vi "ReadMultiTofv2.vi"(6 "Attempts":i32=1, 7 "Relays":tag[](array[tag])=["B/DIO0", "B/DIO1", "B/DIO2", "B/DIO3"], 8 "error in":errorcluster, 10 "I2C Channel":u8=1) -> (0 "error out":errorcluster, 1 "ToF Online":bool[](array[boolean]), 2 "ToF Details":T1[](array[typedef]) {"I2C Slave Address" format="%02x"})   [LabVIEW 2017]
uses:
  <vilib>/myRIO/Common/Instrument Driver Framework/myRIO v1.0/DIO/typedefs/DIO Channels Enum.ctl
  <vilib>/myRIO/Common/Instrument Driver Framework/myRIO v1.0/DIO/typedefs/DIO Channels List.ctl
  <vilib>/myRIO/Common/Instrument Driver Framework/Utilities/typedefs/Generic FPGA Reference.ctl
  <vilib>/myRIO/Common/Instrument Driver Framework/Utilities/typedefs/myRIO v1.0 Reference.ctl
  <vilib>/myRIO/Common/Instrument Driver Framework/Utilities/typedefs/Hardware Version Enum.ctl
  <vilib>/myRIO/Common/Instrument Driver Framework/Utilities/typedefs/myRIO Generic Hardware Reference.ctl
  <vilib>/myRIO/Instrument Drivers/Onboard IO/DIO/typedefs/DIO Reference.ctl
  <vilib>/myRIO/Instrument Drivers/Onboard IO/DIO/DIO.lvlib
  <vilib>/myRIO/Instrument Drivers/Onboard IO/DIO/vis/myRIO DIO Open.xnode
  <vilib>/myRIO/Common/Instrument Driver Framework/myRIO v1.0/DIO/vis/myRIO v1.1 Open DIO.vi
  <vilib>/userdefined/High Color/nirio_resource_hc.ctl
  Sensors/Time of Flight - VL6180/VL6180 Resource.ctl
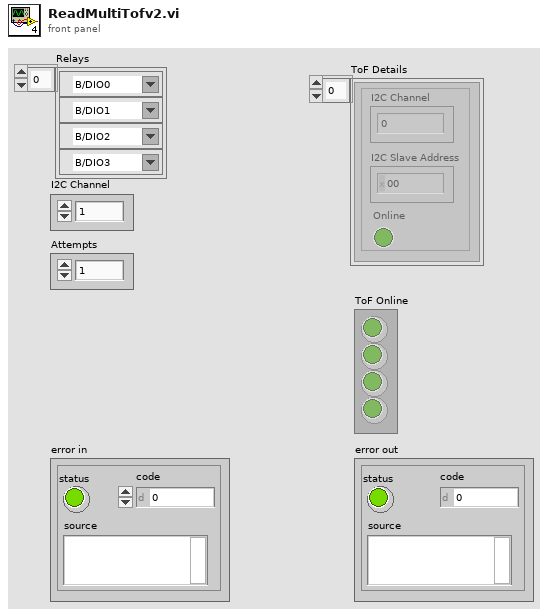
[diagram p1: front panel]
types:
  T1 = typedef "VL6180 Resource.ctl" = cluster{"I2C Channel":u8, "I2C Slave Address":u8, "Online":bool}
  T2 = typedef "DIO.lvlib/DIO Reference.ctl" = cluster{"myRIO Reference":T3, "DIO Channels List":T7}
  T3 = typedef "myRIO Generic Hardware Reference.ctl" = cluster{"myRIO Model":T4, "myRIO Hardware Reference":T5}
  T4 = typedef "Hardware Version Enum.ctl" = enum16{"Unknown", "myRIO-1900", "myRIO-1950", "roboRIO", "NI ELVIS RIO CM", "ELVIS III"}
  T5 = typedef "myRIO v1.0 Reference.ctl" = cluster{"Generic FPGA Reference":T6, "Allow multiple opens":bool}
  T6 = typedef "Generic FPGA Reference.ctl" = refnum<k20>
  T7 = typedef "DIO Channels List.ctl" = T8[]
  T8 = typedef "DIO Channels Enum.ctl" = enum16{"Not Connected", "C/DIO0", "C/DIO1", "C/DIO2", "C/DIO3", "C/DIO4", "C/DIO5", "C/DIO6", "C/DIO7", "A/DIO0", "A/DIO1", "A/DIO2", "A/DIO3", "A/DIO4", "A/DIO5", "A/DIO6", "A/DIO7", "A/DIO8", "A/DIO9", "A/DIO10", "A/DIO11", "A/DIO12", "A/DIO13", "A/DIO14", "A/DIO15", "A/DIO16", "A/DIO17", "A/DIO18", "A/DIO19", "B/DIO0", "B/DIO1", "B/DIO2", "B/DIO3", "B/DIO4", "B/DIO5", "B/DIO6", "B/DIO7", "B/DIO8", "B/DIO9", "B/DIO10", "B/DIO11", "B/DIO12", "B/DIO13", "B/DIO14", "B/DIO15", "B/DIO16", "B/DIO17", "B/DIO18", "B/DIO19", "LED0", "LED1", "LED2", "LED3", "Button0", "DIO/DIO0", "DIO/DIO1", "DIO/DIO2", "DIO/DIO3", "DIO/DIO4", "DIO/DIO5", "DIO/DIO6", "DIO/DIO7", "DIO/DIO8", "DIO/DIO9", "SPI/CS0", "SPI/CS1", "SPI/CS2", "SPI/CS3", "LED RADIO (Green)", "LED RADIO (Red)", "LED COMM (Green)", "LED COMM (Red)", "LED MODE (Green)", "LED MODE (Red)"}
  T9 = typedef "nirio_resource_hc.ctl" = tag
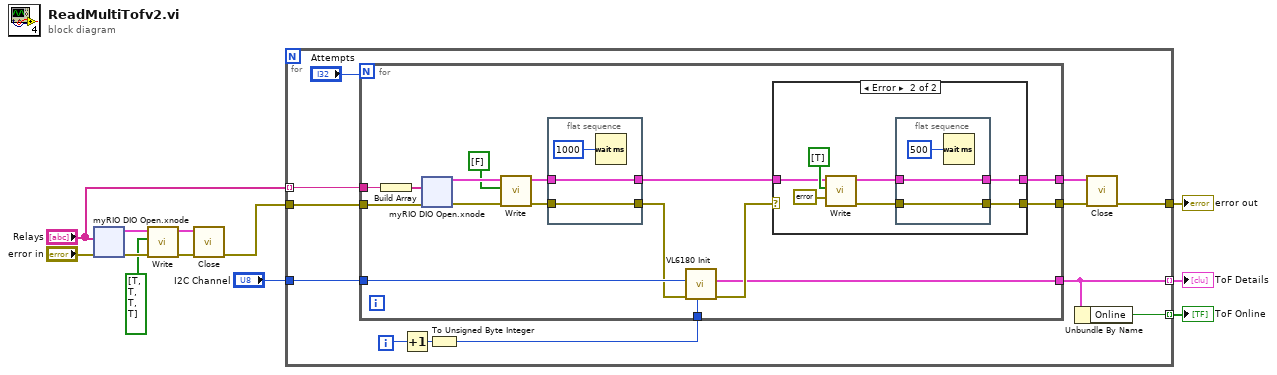
[diagram p0: block diagram]
diagram:
  n1 = xnode "myRIO DIO Open.xnode"("error in (no error)"="error in", "Channel Names"="Relays") -> ("error out"=w6:errorcluster, "DIO Ref Out"=w7:T2)  [unwired: 1 in]
  n2 = call <vilib>:"Write.vi"("error in (no error)"=w6, "Values"=bool[] [TRUE, TRUE, TRUE, TRUE], "DIO Ref In"=w7) -> ("error out"=w3:errorcluster, "DIO Ref Out"=w4:T2)  [unwired: 6 in]
  n3 = call <vilib>:"Close.vi"("error in (no error)"=w3, "DIO Ref In"=w4) -> ("error out"=w2:errorcluster)  [unwired: 9 in]
  n4 = for {
    tunnel: w2 -> [w24]
    tunnel: "Relays" -> [w23] mode=indexing
    tunnel: "I2C Channel" -> [w21]
    tunnel: [w15] -> w11
    tunnel: [w14] -> w10 mode=indexing
    tunnel: [w13] -> w9 mode=indexing
    i -> [w22]
    n5 = Increment(x=w22) -> (x+1=w20:i32)
    n6 = To Unsigned Byte Integer(number=w20) -> (unsigned 8bit integer=w19:u8)
    n7 = for {
      N: "Attempts" -> [_]
      tunnel: w24 -> [w40]
      tunnel: w23 -> [w38]
      tunnel: w21 -> [w34]
      tunnel: w19 -> [w31]
      tunnel: [w27] -> w18
      tunnel: [w26] -> w16
      tunnel: [w25] -> w14
      n8 = Build Array(w38) -> (w39:tag[])
      n9 = xnode "myRIO DIO Open.xnode"("error in (no error)"=w40, "Channel Names"=w39) -> ("error out"=w37:errorcluster, "DIO Ref Out"=w36:T2)  [unwired: 1 in]
      n10 = call <vilib>:"Write.vi"("error in (no error)"=w37, "Values"=bool[] [FALSE], "DIO Ref In"=w36) -> ("error out"=w33:errorcluster, "DIO Ref Out"=w29:T2)  [unwired: 6 in]
      n11 = flat-sequence {
        tunnel: [w54] -> w32
        tunnel: w33 -> [w54]
        tunnel: w29 -> [w53]
        tunnel: [w53] -> w28
        frame #0 {
          n12 = Wait (ms)(milliseconds to wait=u32 1000) -> ()  [unwired: 1 out]
        }
      }
      n13 = call "VL6180 Init.vi"("Change Slave Address"=w31, "Error In"=w32, "I2C Channel"=w34) -> ("Error Out"=w30:errorcluster, "VL6180 Resource"=w25:T1)  [unwired: 6 in, 1 out]
      n14 = case shown="Error" w30 {
        selector: w30 -> [w42 _]
        tunnel: w28 -> [w41 w47]
        tunnel: [w42 w45] -> w26
        tunnel: [w41 w43] -> w27
        frame No Error {
        }
        frame Error {
          n15 = call <vilib>:"Write.vi"("error in (no error)"=errorcluster {"status"=FALSE, "code"=0, "source"=""}, "Values"=bool[] [TRUE], "DIO Ref In"=w47) -> ("error out"=w46:errorcluster, "DIO Ref Out"=w44:T2)  [unwired: 6 in]
          n16 = flat-sequence {
            tunnel: [w51] -> w45
            tunnel: w46 -> [w51]
            tunnel: w44 -> [w50]
            tunnel: [w50] -> w43
            frame #0 {
              n17 = Wait (ms)(milliseconds to wait=u32 500) -> ()  [unwired: 1 out]
            }
          }
        }
      }
    }
    n18 = Unbundle By Name(w14) -> ("Online"=w13:bool)
    n19 = call <vilib>:"Close.vi"("error in (no error)"=w16, "DIO Ref In"=w18) -> ("error out"=w15:errorcluster)  [unwired: 9 in]
  }
  "error out" <- w11
  "ToF Details" <- w10
  "ToF Online" <- w9
